vi "Smite.vi"(8 "Error In":errorcluster, 11 "Graves":refnum<vi>[](array[refnum])) -> (0 "Error Out":errorcluster, 3 "Change Made?":bool)   [LabVIEW 2017, in "Toolkit.lvlib"]
doc: "Changes a grave site (Diagram Disable structure) to the Spirit frame (refactored code) and enables it. In other words, it smites zombie code."
uses:
  Toolkit.lvlib
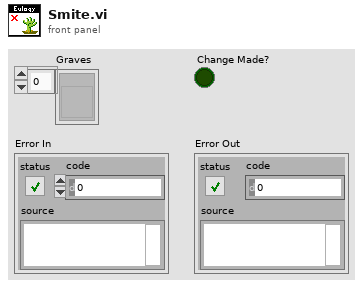
[diagram p1: front panel]
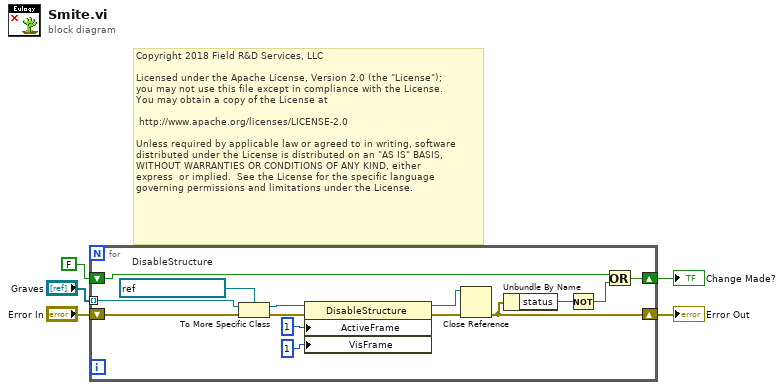
[diagram p0: block diagram]
diagram:
  # "Copyright 2018 Field R&D Services, LLC\n\nLicensed under the Apache License, Version 2.0 (the \"License\");\nyou may not use this file except in compliance with the License.\nYou may obtain a copy of the License at\n\n\thttp://www.apache.org/licenses/LICENSE-2.0\n\nUnless required by applicable law or agreed to in writing, software\ndistributed under the License is distributed on an \"AS IS\" BASIS,\nWITHOUT WARRANTIES OR CONDITIONS OF ANY KIND, either \nexpress  or implied.  See the License for the specific language \ngoverning permissions and limitations under the License."
  n1 = for {
    shift-right: [w8] -> w5
    shift-left: "Error In" -> [w15]
    tunnel: "Graves" -> [w16] mode=indexing
    shift-right: [w18] -> w3
    shift-left: FALSE -> [w19]
    w14 = refnum<vi> refnum  # DisableStructure
    n2 = To More Specific Class(target class=w14, reference=w16, error in=w15) -> (specific class reference=w13:refnum<vi>, error out=w12:errorcluster)
    n3 = property class="DisableStructure"(reference=w13, error in=w12, "ActiveFrame"=i16 1 ("Active Frame"), "VisFrame"=u32 1 ("Visible Frame")) -> (reference out=w9:refnum<vi>, error out=w17:errorcluster)
    n4 = Close Reference(reference=w9, error in (no error)=w17) -> (error out=w8:errorcluster)
    n5 = Unbundle By Name(w8) -> ("status"=w7:bool)
    n6 = Not(x=w7) -> (.not. x?=w6:bool)
    n7 = Or(x=w19, y=w6) -> (x .or. y?=w18:bool)
  }
  "Error Out" <- w5
  "Change Made?" <- w3
